vi "GetConnectionAliasString.vi"(8 "error in (no error)":errorcluster, 11 "EthernetDigitalOutputModbus in":refnum<class "TesteractHAL_DigitalOutput_EthernetModbus.lvclass">=refnum) -> (0 "error out":errorcluster, 2 "Connection Alias":string, 3 "EthernetDigitalOutputModbus out":refnum<class "TesteractHAL_DigitalOutput_EthernetModbus.lvclass">)   [LabVIEW 2017]
uses:
  TesteractHAL_DigitalOutput_EthernetModbus.lvclass
  C:/Program Files (x86)/Testeract/HWLib/HAL/DigitalOutput/TesteractHAL_DigitalOutput.lvlibp/TesteractHAL_DigitalOutput.lvclass
  C:/Program Files (x86)/Testeract/HWLib/HAL/Device/TesteractHAL_Device.lvlibp/TesteractHAL_Device.lvclass
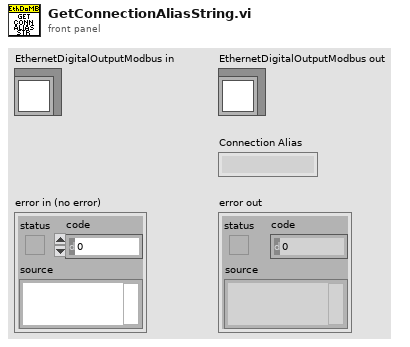
[diagram p1: front panel]
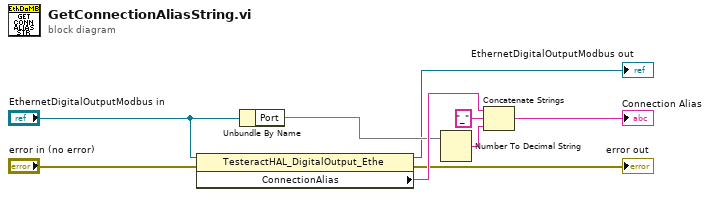
[diagram p0: block diagram]
diagram:
  n1 = property class="TesteractHAL_DigitalOutput_Ethe"(reference="EthernetDigitalOutputModbus in", error in="error in (no error)") -> (reference out=→"EthernetDigitalOutputModbus out":refnum<class "TesteractHAL_DigitalOutput_EthernetModbus.lvclass">, error out=→"error out":errorcluster, "ConnectionAlias"=w7:string)
  n2 = Unbundle By Name("EthernetDigitalOutputModbus in") -> ("Port"=w6)
  n3 = Number To Decimal String(number=w6) -> (decimal integer string=w8:string)  [unwired: 1 in]
  n4 = Concatenate Strings(w7, "_" ("string"), w8) -> (→"Connection Alias":string)
